vi "test Broken.vi"(8 "error in (no error)":errorcluster, 11 "Dummy in":refnum<class "Dummy.lvclass">) -> (0 "error out":errorcluster, 3 "Dummy out":refnum<class "Dummy.lvclass">)   [LabVIEW 2020, in "Dummy.lvclass"]
doc: "Broken test method"
uses:
  Dummy.lvclass
  C:/git/astemes-lunit/source/Core/LUnit Test Case/LUnit Test Case.lvclass
  API/LUnit Test Case/LUnit Test Case.lvclass/LUnit Test Case.ctl
  API/LUnit Test Case/Private/Append Pass Result.vi
  API/LUnit Test Case/LUnit Test Case.lvclass
panel:
  out "x+y":dbl
  in  "x":dbl
  in  "y":dbl
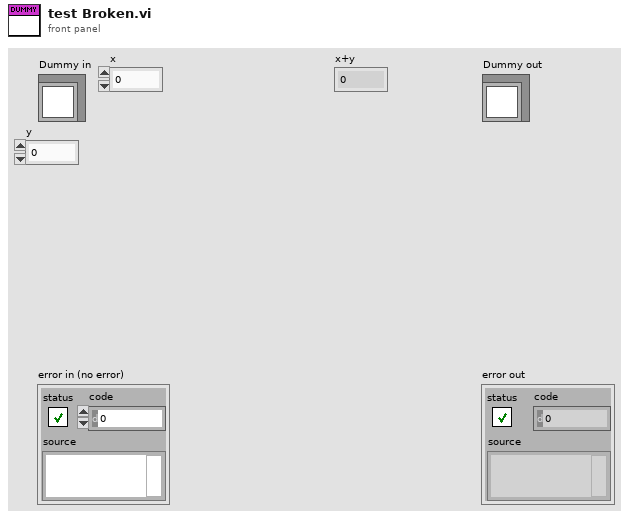
[diagram p1: front panel]
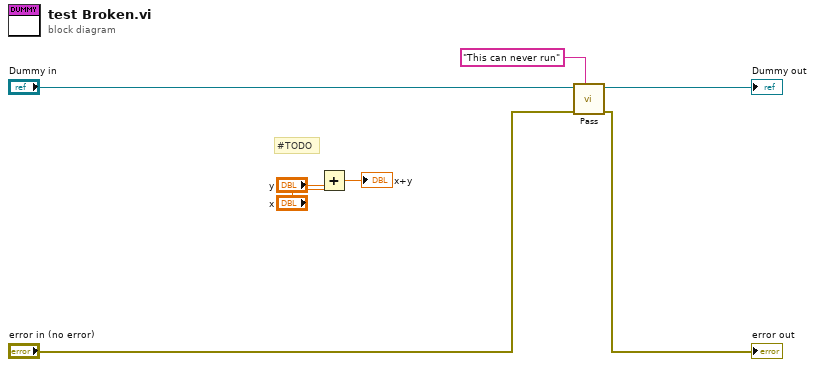
[diagram p0: block diagram]
diagram:
  # "#TODO"
  n1 = Add(x="x", y="y") -> (x+y=→"x+y":dbl)
  n2 = call "Pass.vi"("Description"="This can never run", "error in (no error)"="error in (no error)", "LUnit Test Case In"="Dummy in") -> ("error out"=→"error out":errorcluster, "LUnit Test Case Out"=→"Dummy out":refnum<class "Dummy.lvclass">)  [unwired: 7 in]
